vi "SQL Statement for Sample Descritpion.vi"(4 "error IN":errorcluster, 5 "Layer Weight Array":sgl[](array[numeric]), 6 "VALUES clause IN":string, 7 "INSERT clause IN":string) -> (0 "error OUT":errorcluster, 2 "VALUES clause OUT":string, 3 "INSERT clause OUT":string)   [LabVIEW 2015]
uses:
  BIMS_Collector Globals.vi
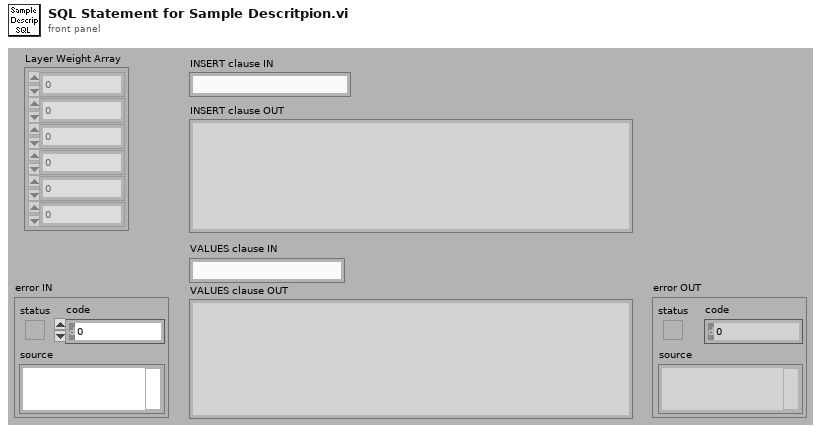
[diagram p1: front panel]
types:
  T1 = cluster{"fiber":string, "denier":string, "pick":string, "weave":string, "finish":string, "ozPerYd2":string, "internal_ID":string, "asset":string}[]
  T2 = cluster{"numOfPlies":i32, "LotNum":string, "RollNum":string}[]
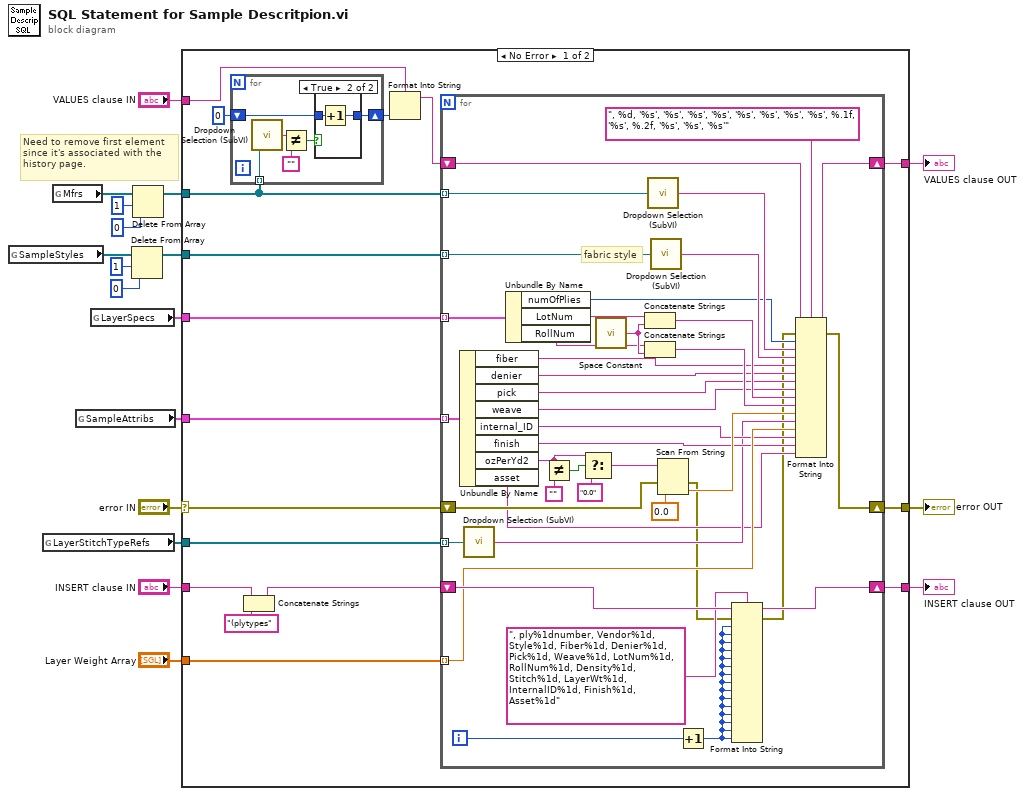
[diagram p0: block diagram]
diagram:
  # "Need to remove first element\nsince it's associated with the \nhistory page."
  n1 = global read "BIMS_Collector Globals.vi" "SampleStyles"() -> (w5:refnum<vi>[])
  n2 = global read "BIMS_Collector Globals.vi" "LayerStitchTypeRefs"() -> (w15:refnum<vi>[])
  n3 = global read "BIMS_Collector Globals.vi" "Mfrs"() -> (w3:refnum<vi>[])
  n4 = global read "BIMS_Collector Globals.vi" "SampleAttribs"() -> (w1:T1)
  n5 = global read "BIMS_Collector Globals.vi" "LayerSpecs"() -> (w10:T2)
  n6 = Delete From Array(array=w5, length=1, index=0) -> (array with subset deleted=w4:refnum<vi>[])  [unwired: 1 out]
  n7 = Delete From Array(array=w3, length=1, index=0) -> (array with subset deleted=w2:refnum<vi>[])  [unwired: 1 out]
  n8 = case shown="No Error" "error IN" {
    selector: "error IN" -> [w24 w88]
    tunnel: [w33 w88] -> w17
    tunnel: "VALUES clause IN" -> [w19 w87]
    tunnel: w2 -> [w23 _]
    tunnel: w4 -> [w32 _]
    tunnel: w1 -> [w31 _]
    tunnel: w15 -> [w30 _]
    tunnel: "INSERT clause IN" -> [w29 w86]
    tunnel: "Layer Weight Array" -> [w28 _]
    tunnel: [w27 w87] -> w12
    tunnel: [w26 w86] -> w11
    tunnel: w10 -> [w25 _]
    frame No Error {
      n9 = for {
        tunnel: w23 -> [w41] mode=indexing
        shift-right: [w36] -> w21
        shift-left: 0 ("index") -> [w37]
        n10 = call "Dropdown Selection (SubVI).vi"("reference"=w41) -> ("element"=w40:string)
        n11 = Not Equal?(x=w40, y="") -> (x != y?=w38:bool)
        n12 = case shown="True" w38 {
          tunnel: w37 -> [w42 w43]
          tunnel: [w42 w44] -> w36
          frame False {
          }
          frame True {
            n13 = Increment(x=w43) -> (x+1=w44:i32)
          }
        }
      }
      n14 = Concatenate Strings(w29, "(plytypes") -> (w35:string)
      n15 = Format Into String(format string=w19, w21) -> (resulting string=w20:string)  [unwired: 2 in, 1 out]
      n16 = for {
        shift-right: [w84] -> w27
        shift-left: w20 -> [w85]
        shift-right: [w81] -> w26
        shift-left: w35 -> [w82]
        tunnel: w28 -> [w76] mode=indexing
        tunnel: w31 -> [w80] mode=indexing
        tunnel: w32 -> [w79] mode=indexing
        tunnel: w25 -> [w77] mode=indexing
        tunnel: w23 -> [w78] mode=indexing
        tunnel: w30 -> [w75] mode=indexing
        shift-right: [w73] -> w33
        shift-left: w24 -> [w74]
        i -> [w83]
        # "fabric style"
        n17 = Unbundle By Name(w80) -> ("fiber"=w63:string, "denier"=w61:string, "pick"=w57:string, "weave"=w62:string, "internal_ID"=w56:string, "finish"=w55:string, "ozPerYd2"=w47:string, "asset"=w52:string)
        n18 = call "Dropdown Selection (SubVI).vi"("reference"=w75) -> ("element"=w54:string)
        n19 = Unbundle By Name(w77) -> ("numOfPlies"=w58:i32, "LotNum"=w66:string, "RollNum"=w67:string)
        n20 = Not Equal?(x=w47, y="") -> (x != y?=w48:bool)
        n21 = Select(t=w47, s=w48, f="0.0") -> (s? t:f=w46:string)
        n22 = call <vilib>:"Space Constant.vi"() -> ("String"=w68:string)
        n23 = Concatenate Strings(w66, w68) -> (w70:string)
        n24 = Concatenate Strings(w67, w68) -> (w69:string)
        n25 = call "Dropdown Selection (SubVI).vi"("reference"=w78) -> ("element"=w64:string)
        n26 = call "Dropdown Selection (SubVI).vi"("reference"=w79) -> ("element"=w65:string)
        n27 = Scan From String(input string=w46, error in=w74, default 1=sgl 0.0 ("default value 1")) -> (error out=w51:errorcluster, output 1=w60:sgl)  [unwired: 2 in, 2 out]
        n28 = Increment(x=w83) -> (x+1=w53:i32)
        n29 = Format Into String(format string=", ply%1dnumber, Vendor%1d, Style%1d, Fiber%1d, Denier%1d, Pick%1d, Weave%1d, LotNum%1d, RollNum%1d, Density%1d, Stitch%1d, LayerWt%1d, InternalID%1d, Finish%1d, Asset%1d", initial string=w82, error in=w51, w53, w53, w53, w53, w53, w53, w53, w53, w53, w53, w53, w53, w53, w53, w53) -> (resulting string=w81:string, error out=w50:errorcluster)
        n30 = Format Into String(format string=", %d, '%s', '%s', '%s', '%s', '%s', '%s', '%s', '%s', %.1f, '%s', %.2f, '%s', '%s', '%s'", initial string=w85, error in=w50, w58, w64, w65, w63, w61, w57, w62, w70, w69, w60, w54, w76, w56, w55, w52) -> (resulting string=w84:string, error out=w73:errorcluster)
      }
    }
    frame Error {
    }
  }
  "error OUT" <- w17
  "VALUES clause OUT" <- w12
  "INSERT clause OUT" <- w11
